vi "LWXPS_Example_APIListGet.vi"() -> ()   [LabVIEW 2013]
panel:
  out "XPS Error String":string
  out "API Method List":string
  out "Error out":errorcluster caption="error out"
  out "Error code":i32
  in  "Instrument Key IN":string
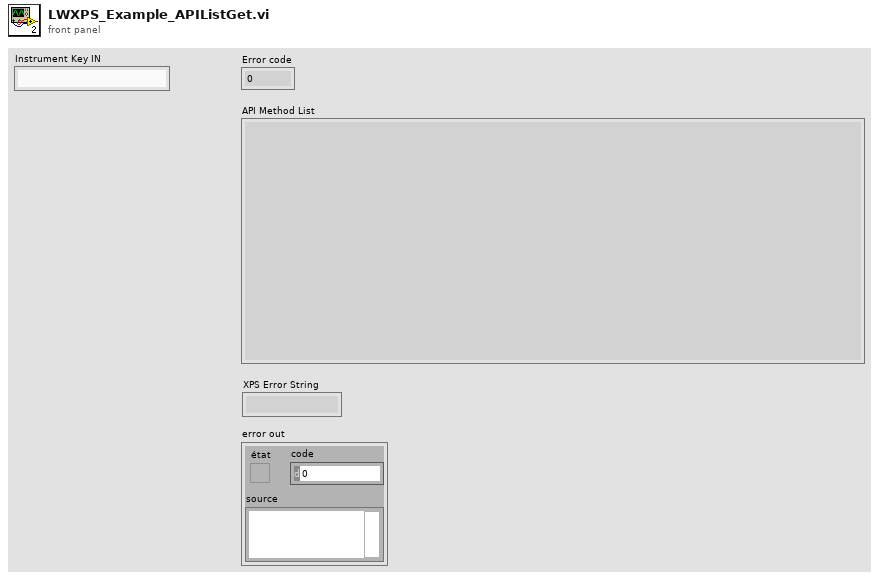
[diagram p1: front panel]
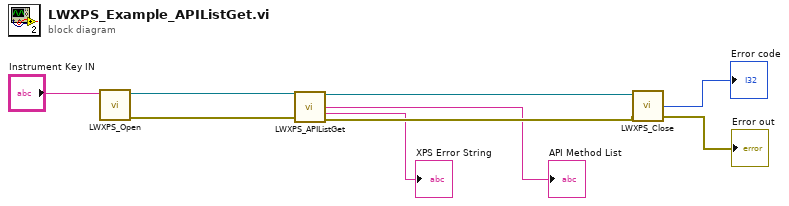
[diagram p0: block diagram]
diagram:
  n1 = call "LWXPS_Open.vi"("Instrument Key IN"="Instrument Key IN") -> ("error out"=w7:errorcluster, "CommandInterfaceXPS.XPS"=w8:refnum<k24>)  [unwired: 3 in, 2 out]
  n2 = call "LWXPS_APIListGet.vi"("XPS Reference IN"=w8, "LabVIEW error IN"=w7) -> ("CommandInterfaceXPS.XPS"=w6:refnum<k24>, "API Method List"=→"API Method List":string, "XPS Error String"=→"XPS Error String":string, "LabVIEW error OUT"=w5:errorcluster)  [unwired: 9 in, 1 out]
  n3 = call "LWXPS_Close.vi"("error in (no error)"=w5, "XPS Reference"=w6) -> ("Error out"=→"Error out":errorcluster, "Error code"=→"Error code":i32)  [unwired: 2 in]
